vi "Std_Bus_ReadValue.vi"(0 "ILabVIEW In":refnum<k24>, 1 "DeviceType":i32(ring) items=["Controller", "RUI", "PC", "CommsCard"], 2 "Zone":i32, 3 "ParameterID":i32, 4 "InstanceId":i32, 5 "error in (no error)":errorcluster, 6 "TemperatureUnits":u8(ring) items=["Degrees F", "Degrees C"]) -> (14 "ILabVIEW Out":refnum<k24>, 17 "Value Out":string, 19 "error out":errorcluster)   [LabVIEW 2018]
doc: "This VI is used to read a parameter specified by the user. Refer to users manual (CIP) Class Instance Attribute column for <B>Parameter ID</B> values.\n\n<B>DeviceType</B> is the type of device being connected to. \nThe selections are:\n <B>Control</B> - This will be one of the following Watlow controllers (PM Family, RM Family, ST Family and F4T)\n<B> RUI</B> - This will be any Watlow Remote User Interface\n<B> PC</B> - Not used at this time\n<B> CommsCard</B> Not used at this time\n\n<B>Zone</B> is the logical address. Range 1-17.\n\nThe <B>Instance</B> defines the occurrence of the feature.\nExample:\nInput 1 - <B>Instance 1</B>\nInput 2 - <B>Instance 2</B>\nAlarm 1 - <B>Instance 1</B>\nAlarm 2 - <B>Instance 2</B>\nOutput 1 - <B>Instance 1</B>\nOutput 2 - <B>Instance 2</B>\nDIO1 (Output 5) - <B>Instance 5</B>\nDIO2 (Output 6) - <B>Instance 6</B>\netc."
uses:
  C:/RageATE/Instruments/Ess Temp Plate/LabView Driver/Public/Watbus.dll
  Watbus.dll
panel:
  # "Std Bus Read"
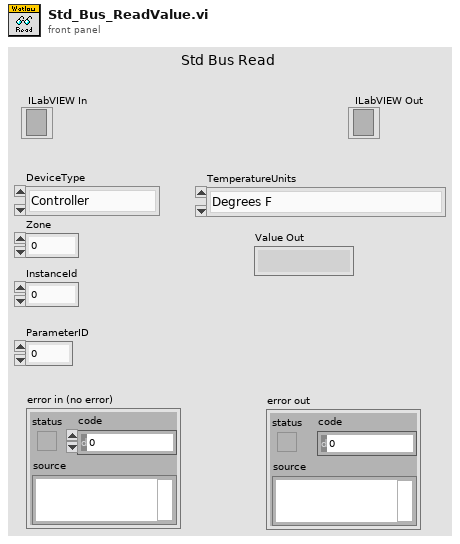
[diagram p1: front panel]
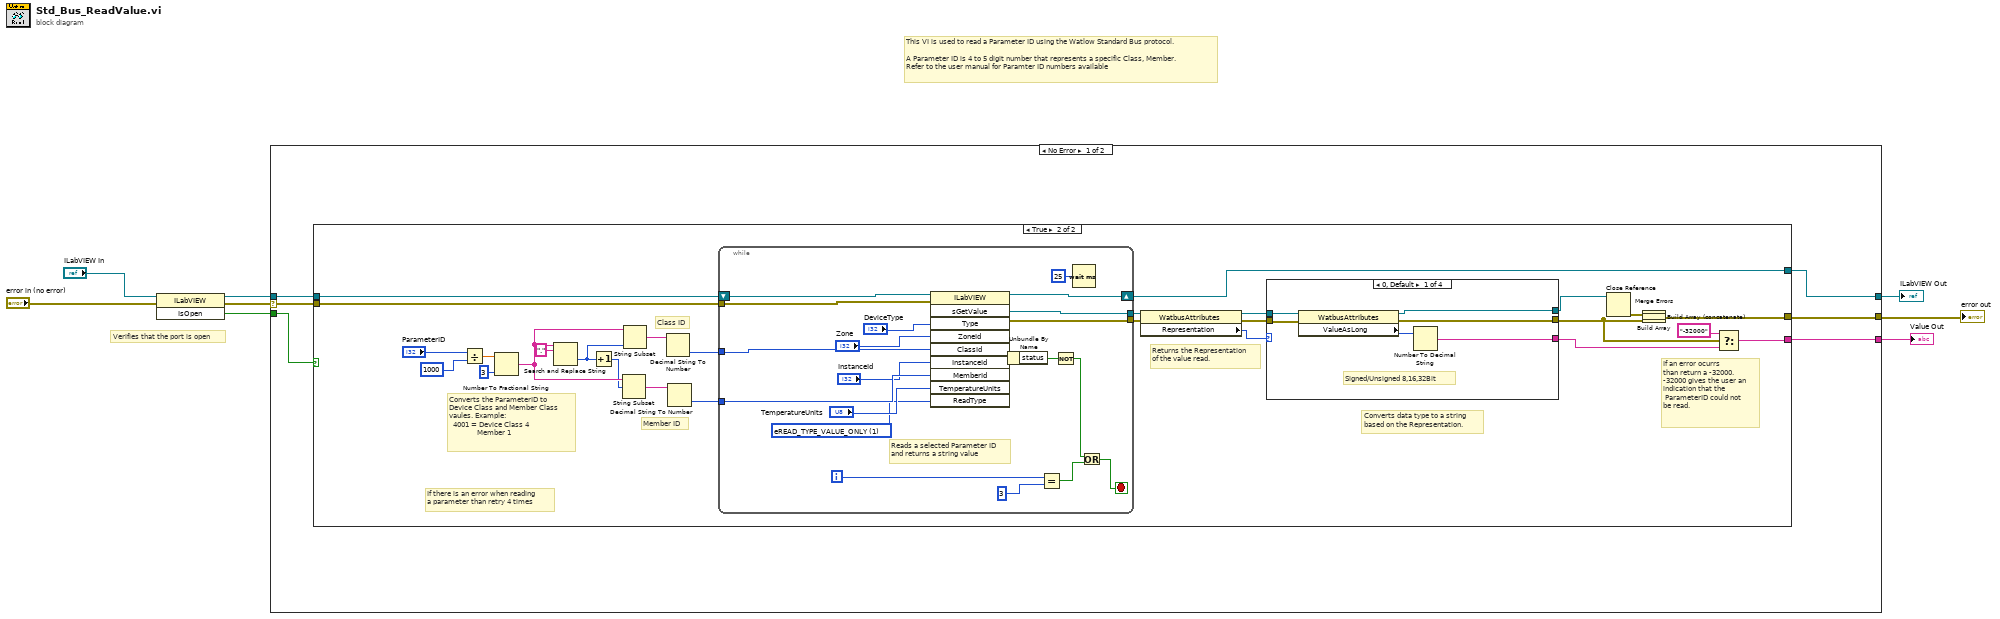
[diagram p0: block diagram]
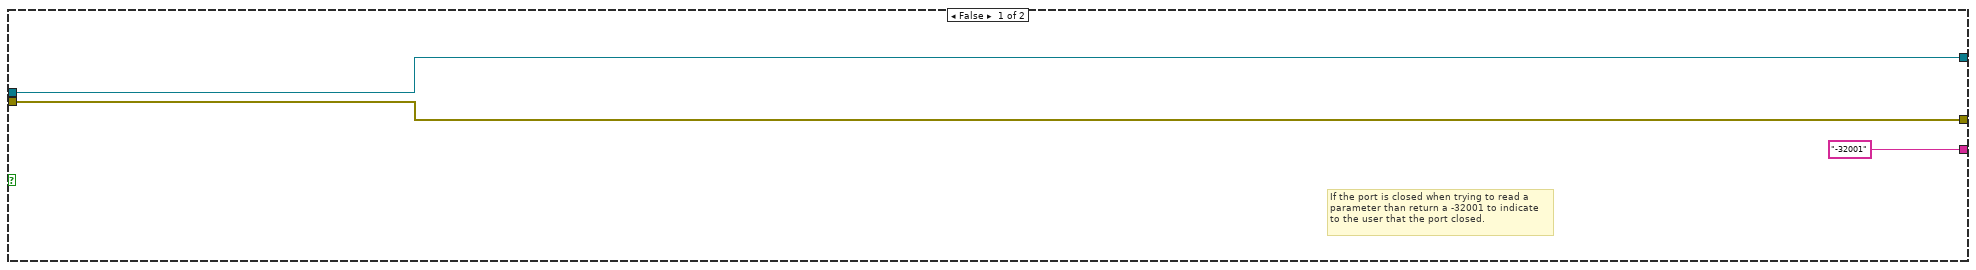
[diagram p2: hidden frame]
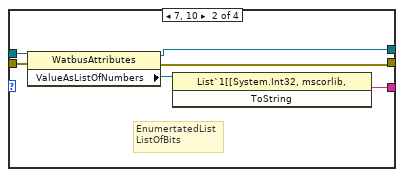
[diagram p3: hidden frame]
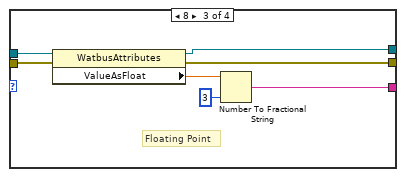
[diagram p4: hidden frame]
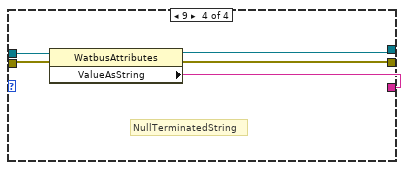
[diagram p5: hidden frame]
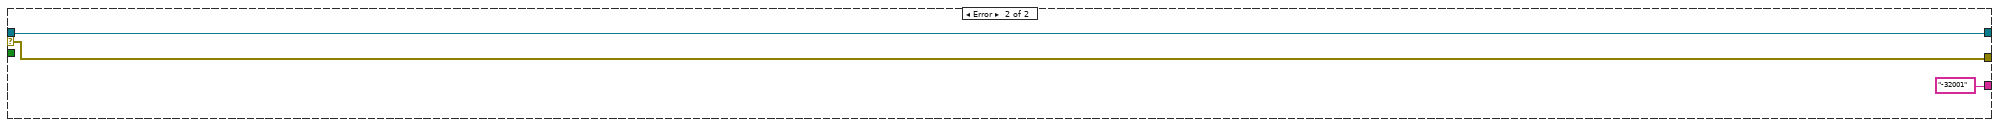
[diagram p6: hidden frame]
diagram:
  # "Verifies that the port is open"
  # "This VI is used to read a Parameter ID using the Watlow Standard Bus protocol.\n\nA Parameter ID is 4 to 5 digit number that represents a specific Class, Member.\nRefer to the user manual for Paramter ID numbers available"
  n1 = invoke class="ILabVIEW" method="IsOpen"(reference="ILabVIEW In", error in="error in (no error)") -> (reference out=w6:refnum<k24>, error out=w5:errorcluster, "IsOpen"=w3:bool)  [unwired: 1 in]
  n2 = case shown="No Error" w5 {
    selector: w5 -> [w10 w92]
    tunnel: [w14 "-32001" ("ValueAsString")] -> w8
    tunnel: [w13 w90] -> w1
    tunnel: w6 -> [w12 w90]
    tunnel: [w11 w92] -> w7
    tunnel: w3 -> [w9 _]
    frame No Error {
      n3 = case shown="True" w9 {
        tunnel: ["-32001" ("ValueAsString") w24] -> w14
        tunnel: w12 -> [w15 w29]
        tunnel: w10 -> [w16 w28]
        tunnel: [w16 w20] -> w11
        tunnel: [w15 w27] -> w13
        frame False {
          # "If the port is closed when trying to read a\nparameter than return a -32001 to indicate\nto the user that the port closed."
        }
        frame True {
          # "If there is an error when reading\na parameter than retry 4 times"
          # "Returns the Representation\nof the value read."
          # "If an error ocurrs\nthan return a -32000.\n-32000 gives the user an\nindication that the\n ParameterID could not \nbe read."
          # "Converts the ParameterID to\nDevice Class and Member Class\nvaules. Example:\n  4001 = Device Class 4\n              Member 1"
          # "Class ID"
          # "Member ID"
          # "Converts data type to a string \nbased on the Representation."
          n4 = Divide(x="ParameterID", y=1000) -> (x/y=w34:dbl)
          n5 = Number To Fractional String(number=w34, precision (6)=i16 3) -> (F-format string=w39:string)  [unwired: 2 out]
          n6 = Search and Replace String(input string=w39, search string=".") -> (offset past replacement=w40:i32)  [unwired: 1 in, 8 out]
          n7 = Increment(x=w40) -> (x+1=w37:i32)
          n8 = String Subset(string=w39, offset (0)=w37) -> (substring=w38:string)  [unwired: 1 out]
          n9 = String Subset(string=w39, length (rest)=w40) -> (substring=w41:string)  [unwired: 1 out]
          n10 = Decimal String To Number(string=w41) -> (number=w31:i32)  [unwired: 3 out]
          n11 = Decimal String To Number(string=w38) -> (number=w30:i32)  [unwired: 3 out]
          n12 = while {
            tunnel: [w65] -> w45
            tunnel: w31 -> [w64]
            tunnel: w30 -> [w63]
            shift-right: [w60] -> w27
            shift-left: w29 -> [w62]
            tunnel: w28 -> [w61]
            tunnel: [w56] -> w46
            i -> [w52]
            stop <- w53 stop-if-true
            w47 = u8 1 items=["eREAD_TYPE_VALUE_ONLY"=1, "eREAD_TYPE_VALUE_AND_ATTRIBUTES"=2] ("ReadType")
            # "Reads a selected Parameter ID\nand returns a string value"
            n13 = invoke class="ILabVIEW" method="sGetValue"(reference=w62, error in=w61, "Type"="DeviceType", "ZoneId"="Zone", "ClassId"=w64, "InstanceId"="InstanceId", "MemberId"=w63, "TemperatureUnits"="TemperatureUnits", "ReadType"=w47) -> (reference out=w60:refnum<k24>, error out=w56:errorcluster, "sGetValue"=w65:refnum<k24>)  [unwired: 1 in, 7 out]
            n14 = Unbundle By Name(w56) -> ("status"=w55:bool)
            n15 = Equal?(x=w52, y=3) -> (x = y?=w51:bool)
            n16 = Not(x=w55) -> (.not. x?=w54:bool)
            n17 = Wait (ms)(milliseconds to wait=u32 25) -> ()  [unwired: 1 out]
            n18 = Or(x=w54, y=w51) -> (x .or. y?=w53:bool)
          }
          n19 = property class="WatbusAttributes"(reference=w45, error in=w46) -> (reference out=w44:refnum<k24>, error out=w42:errorcluster, "Representation"=w43:i32)
          n20 = case shown="0, Default" w43 {
            tunnel: w44 -> [w71 w77 w84 w89]
            tunnel: [w69 w75 w82 w86] -> w25
            tunnel: w42 -> [w68 w74 w80 w88]
            tunnel: [w67 w73 w79 w87] -> w21
            tunnel: [w66 w72 w78 w85] -> w23
            frame 0, Default {
              # "Signed/Unsigned 8,16,32Bit"
              n21 = property class="WatbusAttributes"(reference=w71, error in=w68) -> (reference out=w66:refnum<k24>, error out=w67:errorcluster, "ValueAsLong"=w70:i64)
              n22 = Number To Decimal String(number=w70) -> (decimal integer string=w69:string)  [unwired: 1 out]
            }
            frame 7, 10 {
              # "EnumertatedList\nListOfBits"
              n23 = property class="WatbusAttributes"(reference=w77, error in=w74) -> (reference out=w72:refnum<k24>, error out=w73:errorcluster, "ValueAsListOfNumbers"=w76:refnum<k24>)
              n24 = invoke class="List`1[[System.Int32, mscorlib," method="ToString"(reference=w76) -> ("ToString"=w75:string)  [unwired: 2 in, 2 out]
            }
            frame 8 {
              # "Floating Point"
              n25 = property class="WatbusAttributes"(reference=w84, error in=w80) -> (reference out=w78:refnum<k24>, error out=w79:errorcluster, "ValueAsFloat"=w83:sgl)
              n26 = Number To Fractional String(number=w83, precision (6)=i16 3) -> (F-format string=w82:string)  [unwired: 2 out]
            }
            frame 9 {
              # "NullTerminatedString"
              n27 = property class="WatbusAttributes"(reference=w89, error in=w88) -> (reference out=w85:refnum<k24>, error out=w87:errorcluster, "ValueAsString"=w86:string)
            }
          }
          n28 = Close Reference(reference=w23) -> (error out=w22:errorcluster)  [unwired: 1 in]
          n29 = Build Array(w22, w21) -> (w19:errorcluster[])
          n30 = Build Array (concatenate)(w19) -> (w18:errorcluster[])
          n31 = Merge Errors(w18) -> (w20:errorcluster)
          n32 = Select(t="-32000" ("ValueAsString"), s=w21, f=w25) -> (s? t:f=w24:string)
        }
      }
    }
    frame Error {
    }
  }
  "error out" <- w7
  "Value Out" <- w8
  "ILabVIEW Out" <- w1
